vi "LockinDAQ.setAIconfig.vi"(8 "error in (no error)":errorcluster, 9 "Simulation mode":T1, 10 "AI Configuration":T2 {"input terminal configuration" items=["default"=-1, "RSE"=10083, "NRSE"=10078, "Differential"=10106, "Pseudodifferential"=12529]; "AI.Coupling" items=["AC"=10045, "DC"=10050, "GND"=10066]}, 11 "LockinDAQ":refnum<class "LockinDAQ.lvclass">) -> (0 "error out":errorcluster, 3 "LockinDAQ out":refnum<class "LockinDAQ.lvclass">)   [LabVIEW 2020, in "LockinDAQ.lvclass"]
doc: "---------------------------------------------------------------\nJKI State Machine Objects™\nhttp://jki.net/state-machine-objects/\nCopyright (C) 2005-2015, JKI <info@jki.net>\nALL RIGHTS RESERVEDJKI State Machine Objects (SMO) 1.0.0.4\nJKI - JKI\nCopyright (c) 2015, JKI"
uses:
  LockinDAQ.lvclass
  Typedefs/AI.config-array.ctl
  Typedefs/AI.config-cluster.ctl
  Typedefs/AI.coupling-enum.ctl
  Typedefs/446xAI-enum.ctl
  Typedefs/DAQType-enum.ctl
  LockinDAQ.lvclass/LockinDAQ.ctl
  Typedefs/AI Simulation-enum.ctl
panel:
  # "For instructions on how to use the JKI State Machine Objects, examples and video tutorials, visit:\nhttp://jki.net/state-machine-objects/\n\nJKI State Machine Objects™\nhttp://jki.net/state-machine-objects/\nCopyright (C) 2005-2015, JKI <info@jki.net>\nALL RIGHTS RESERVED"
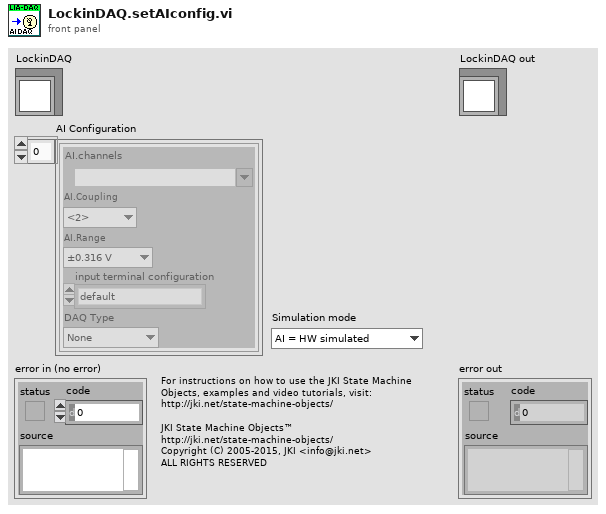
[diagram p1: front panel]
types:
  T1 = typedef "LockinDAQ.lvclass/AI Simulation-enum.ctl" = enum16{"AI = HW simulated", "AI = noise*AO", "AI = waveguide"}
  T2 = typedef "LockinDAQ.lvclass/AI.config-array.ctl" = T3[]
  T3 = typedef "LockinDAQ.lvclass/AI.config-cluster.ctl" = cluster{"AI.channels":tag, "AI.Coupling":T4, "AI.Range":T5, "input terminal configuration":i32, "DAQ Type":T6}
  T4 = typedef "LockinDAQ.lvclass/AI.coupling-enum.ctl" = u16
  T5 = typedef "LockinDAQ.lvclass/446xAI-enum.ctl" = enum16{"±0.316 V", "±1.00 V", "±3.16 V", "±10.0 V", "±31.6 V", "±42.4 V"}
  T6 = typedef "LockinDAQ.lvclass/DAQType-enum.ctl" = enum16{"None", "USB 4431", "PXI 446x"}
  T7 = cluster{"AI Configuration":T2, "Simulation mode":T1}
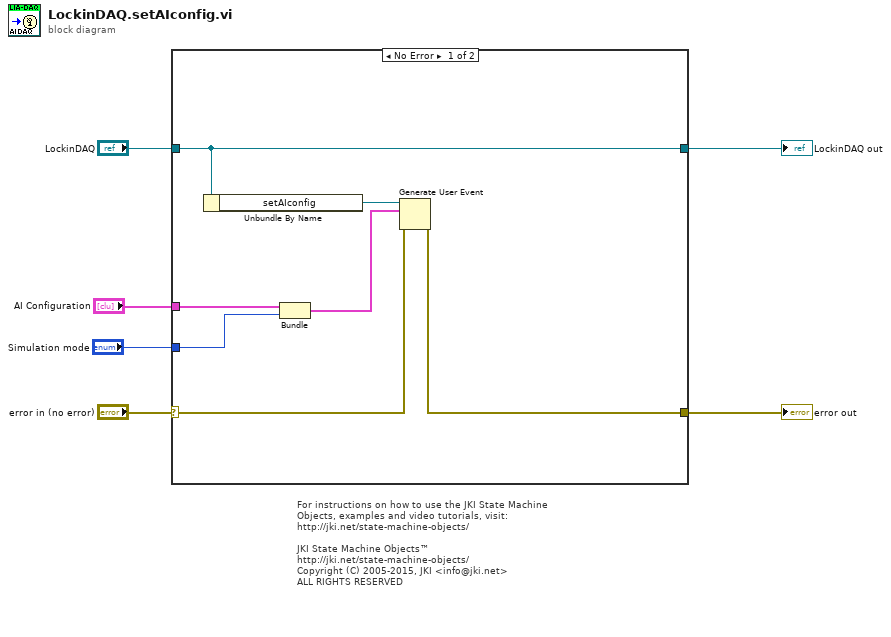
[diagram p0: block diagram]
diagram:
  # "For instructions on how to use the JKI State Machine Objects, examples and video tutorials, visit:\nhttp://jki.net/state-machine-objects/\n\nJKI State Machine Objects™\nhttp://jki.net/state-machine-objects/\nCopyright (C) 2005-2015, JKI <info@jki.net>\nALL RIGHTS RESERVED"
  n1 = case shown="No Error" "error in (no error)" {
    selector: "error in (no error)" -> [w13 w15]
    tunnel: [w11 w15] -> w5
    tunnel: [w10 w14] -> w6
    tunnel: "LockinDAQ" -> [w10 w14]
    tunnel: "AI Configuration" -> [w9 _]
    tunnel: "Simulation mode" -> [w7 _]
    frame No Error {
      n2 = Unbundle By Name(w10) -> ("setAIconfig"=w12:refnum<user-event>)
      n3 = Bundle("AI Configuration"=w9, "Simulation mode"=w7) -> (w8:T7)  [unwired: 1 in]
      n4 = Generate User Event(user event=w12, event data cluster=w8, error in=w13) -> (error out=w11:errorcluster)  [unwired: 1 in, 1 out]
    }
    frame Error {
    }
  }
  "error out" <- w5
  "LockinDAQ out" <- w6
